vi "Copy Config Converter.vi"(11 "error in (no error)":errorcluster) -> (4 "path":path, 15 "error out":errorcluster)   [LabVIEW 2013, in "AIT 664 Custom Device.lvlib"]
doc: "Find and copy the convert.exe application to convert the .xml file to .hex file."
uses:
  AIT 664 Custom Device.lvlib
  <vilib>/Utility/sysdir.llb/System Directory Type.ctl
panel:
  out "Chosen Folder":string
  out "folder names":string[](array[string])
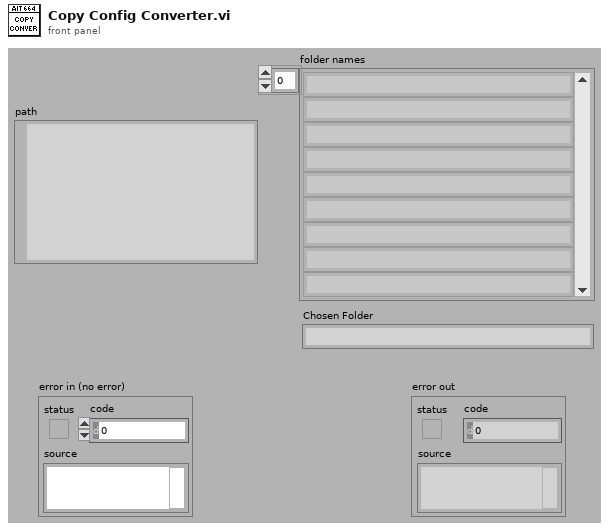
[diagram p1: front panel]
types:
  T1 = typedef "System Directory Type.ctl" = i32
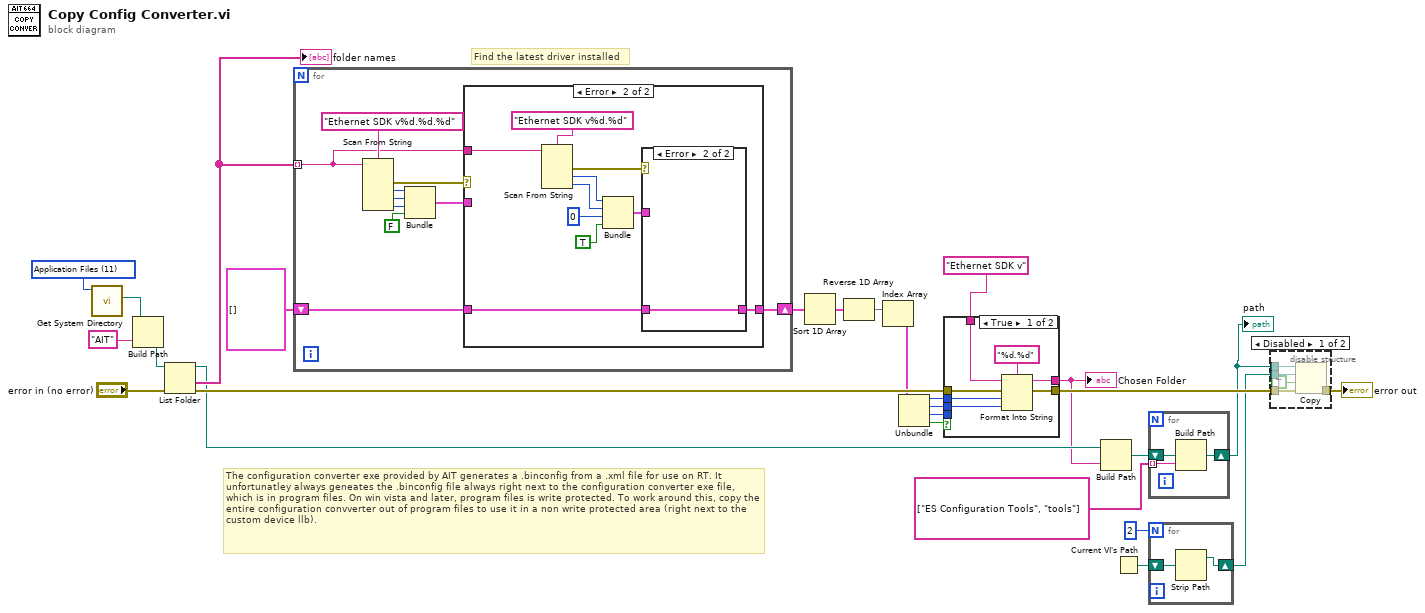
[diagram p0: block diagram]
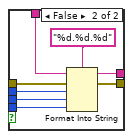
[diagram p3: hidden frame]
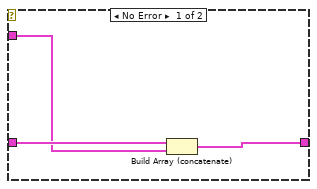
[diagram p4: hidden frame]
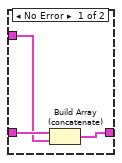
[diagram p5: hidden frame]
diagram:
  w2 = T1 11 items=["User Home"=0, "User Desktop"=1, "User Documents"=2, "User Application Data"=3, "User Preferences"=4, "User Temporary"=5, "Public Documents"=6, "Public Application Data"=7, "Public Preferences"=8, "Public Cache"=13, "System Core Libraries"=9, "System Installed Libraries"=10, "Application Files"=11, "Boot Volume Root"=12] ("system directory type")
  # "The configuration converter exe provided by AIT generates a .binconfig from a .xml file for use on RT. It unfortunatley always geneates the .binconfig file always right next to the configuration converter exe file, which is in program files. On win vista and later, program files is write protected. To work around this, copy the entire configuration convverter out of program files to use it in a non write protected area (right next to the custom device llb)."
  # "Find the latest driver installed"
  n1 = call <vilib>:"Get System Directory.vi"("system directory type"=w2) -> ("system directory"=w3:path)  [unwired: 10 in]
  n2 = Build Path(base path=w3, name or relative path="AIT") -> (appended path=w7:path)
  n3 = List Folder(path=w7, error in="error in (no error)") -> (path out=w15:path, folder names=w25:string[], error out=w20:errorcluster)  [unwired: 2 in, 1 out]
  "folder names" <- w25
  n4 = for {
    tunnel: w25 -> [w28] mode=indexing
    shift-right: [w30] -> w18
    shift-left: cluster{i32, i32, i32, bool}[] [] -> [w32]
    n5 = Scan From String(format string="Ethernet SDK v%d.%d.%d", input string=w28) -> (error out=w33:errorcluster, output 1=w35:i32, output 2=w34:i32, output 3=w37:i32)  [unwired: 5 in, 2 out]
    n6 = Bundle(w35, w34, w37, FALSE) -> (w31:cluster{i32, i32, i32, bool})  [unwired: 1 in]
    n7 = case shown="Error" w33 {
      tunnel: w32 -> [w40 w42]
      tunnel: w31 -> [w38 _]
      tunnel: [w39 w41] -> w30
      tunnel: w28 -> [_ w43]
      frame No Error {
        n8 = Build Array (concatenate)(w40, w38) -> (w39:cluster{i32, i32, i32, bool}[])
      }
      frame Error {
        n9 = Scan From String(format string="Ethernet SDK v%d.%d", input string=w43) -> (error out=w49:errorcluster, output 1=w48:i32, output 2=w47:i32)  [unwired: 4 in, 2 out]
        n10 = Bundle(w48, w47, 0, TRUE) -> (w45:cluster{i32, i32, i32, bool})  [unwired: 1 in]
        n11 = case shown="Error" w49 {
          tunnel: w42 -> [w53 w54]
          tunnel: w45 -> [w52 _]
          tunnel: [w51 w54] -> w41
          frame No Error {
            n12 = Build Array (concatenate)(w53, w52) -> (w51:cluster{i32, i32, i32, bool}[])
          }
          frame Error {
          }
        }
      }
    }
  }
  n13 = Sort 1D Array(array=w18) -> (sorted array=w24:cluster{i32, i32, i32, bool}[])
  n14 = Reverse 1D Array(array=w24) -> (reversed array=w17:cluster{i32, i32, i32, bool}[])
  n15 = Index Array(array=w17) -> (element=w6:cluster{i32, i32, i32, bool})  [unwired: 1 in]
  n16 = Unbundle(w6) -> (w23:i32, w22:i32, w21:i32, w5:bool)
  n17 = case shown="True" w5 {
    tunnel: w23 -> [w60 w68]
    tunnel: w22 -> [w59 w67]
    tunnel: w21 -> [_ w66]
    tunnel: w20 -> [w58 w65]
    tunnel: "Ethernet SDK v" ("format string") -> [w57 w64]
    tunnel: [w56 w63] -> w4
    tunnel: [w55 w62] -> w12
    frame True {
      n18 = Format Into String(format string="%d.%d", initial string=w57, error in=w58, w60, w59) -> (resulting string=w56:string, error out=w55:errorcluster)
    }
    frame False {
      n19 = Format Into String(format string="%d.%d.%d", initial string=w64, error in=w65, w68, w67, w66) -> (resulting string=w63:string, error out=w62:errorcluster)
    }
  }
  "Chosen Folder" <- w4
  n20 = Build Path(base path=w15, name or relative path=w4) -> (appended path=w14:path)
  n21 = Current VI's Path() -> (path=w11:path)
  n22 = for {
    tunnel: string[] ["ES Configuration Tools", "tools"] -> [w71] mode=indexing
    shift-right: [w70] -> w1
    shift-left: w14 -> [w72]
    n23 = Build Path(base path=w72, name or relative path=w71) -> (appended path=w70:path)
  }
  "path" <- w1
  n24 = for {
    N: 2 -> [_]
    shift-right: [w73] -> w9
    shift-left: w11 -> [w74]
    n25 = Strip Path(path=w74) -> (stripped path=w73:path)  [unwired: 1 out]
  }
  n26 = disable-structure shown="Disabled" {
    disable-tunnel: w12 -> [w79 _]
    disable-tunnel: w1 -> [w78 _]
    disable-tunnel: w9 -> [w77 _]
    disable-tunnel: [w76 _] -> w8
    frame Disabled {
      n27 = Copy(8:w79, 9:TRUE ("overwrite (F)"), 10:w77, 11:w78) -> (0:w76:errorcluster)  [unwired: 1 in, 2 out]
    }
    frame Enabled {
    }
  }
  "error out" <- w8
